vi "W_Phi.vi"(9 "Radio":ext, 10 "left motor ccw velocity (rad/s)":dbl, 11 "right motor ccw velocity (rad/s)":dbl) -> (3 "Array out":ext[](array[numeric]))   [LabVIEW 2011]
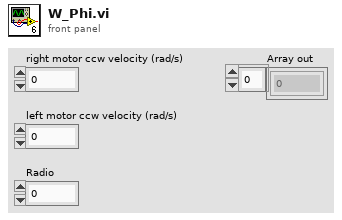
[diagram p1: front panel]
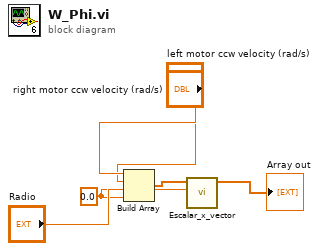
[diagram p0: block diagram]
diagram:
  w1 = 0.0 ("element")
  n1 = Build Array("right motor ccw velocity (rad/s)", "left motor ccw velocity (rad/s)", w1, w1) -> (w4:dbl[])
  n2 = call "Escalar_x_vector.vi"("Numeric"="Radio", "Array in"=w4) -> ("Array out"=→"Array out":ext[])  [unwired: 9 in]
